vi "CleanReplyPi.vi"(10 "text read":string, 11 "Console in":string) -> (3 "String out":string)   [LabVIEW 2019]
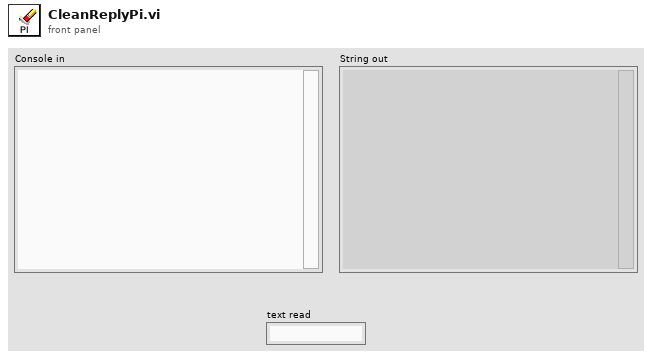
[diagram p1: front panel]
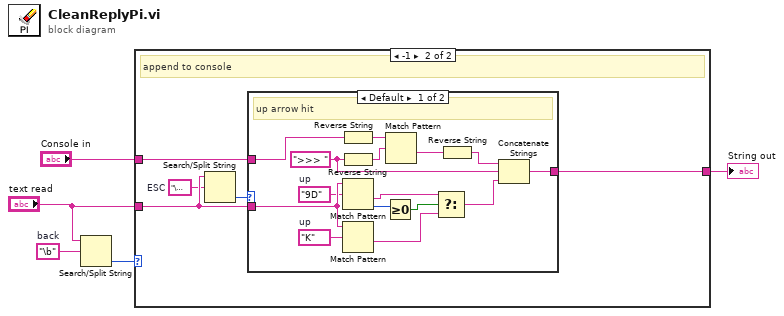
[diagram p0: block diagram]
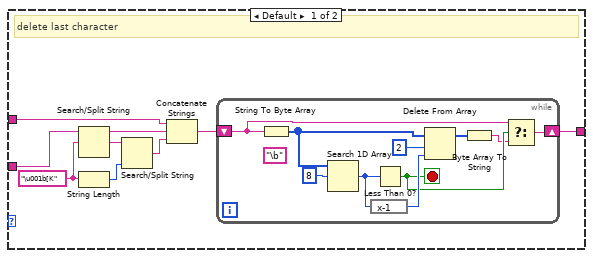
[diagram p2: hidden frame]
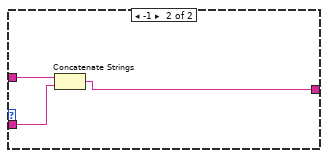
[diagram p3: hidden frame]
diagram:
  w2 = "\b"  # back
  n1 = Search/Split String(string="text read", search string/char (-)=w2) -> (offset of match=w5:i32)  [unwired: 1 in, 2 out]
  n2 = case shown="-1" w5 {
    tunnel: "text read" -> [w12 w27]
    tunnel: "Console in" -> [w14 w29]
    tunnel: [w13 w28] -> w1
    frame Default {
      w9 = "\u001b[K"
      # "delete last character"
      n3 = Search/Split String(string=w12, search string/char (-)=w9) -> (substring before match=w6:string, match + rest of string=w8:string)  [unwired: 1 in, 1 out]
      n4 = String Length(string=w9) -> (length=w10:i32)
      n5 = Search/Split String(string=w8, offset (0)=w10) -> (match + rest of string=w11:string)  [unwired: 1 in, 2 out]
      n6 = Concatenate Strings(w14, w6, w11) -> (w7:string)
      n7 = while {
        shift-right: [w15] -> w13
        shift-left: w7 -> [w17]
        stop <- w18 stop-if-true
        (unwired) "\b"
        n8 = String To Byte Array(string=w17) -> (unsigned byte array=w23:u8[])
        n9 = Search 1D Array(1D array=w23, element=u8 8) -> (index of element=w19:i32)  [unwired: 1 in]
        n10 = expression code="x-1"(w19) -> (w21:i32)
        n11 = Less Than 0?(x=w19) -> (x < 0?=w18:bool)
        n12 = Delete From Array(array=w23, length=2, index=w21) -> (array with subset deleted=w20:u8[])  [unwired: 1 out]
        n13 = Byte Array To String(unsigned byte array=w20) -> (string=w16:string)
        n14 = Select(t=w17, s=w18, f=w16) -> (s? t:f=w15:string)
      }
    }
    frame -1 {
      w25 = "\u001b"  # ESC
      # "append to console"
      n15 = Search/Split String(string=w27, search string/char (-)=w25) -> (offset of match=w26:i32)  [unwired: 1 in, 2 out]
      n16 = case shown="Default" w26 {
        tunnel: w29 -> [w44 w47]
        tunnel: [w43 w46] -> w28
        tunnel: w27 -> [w42 w45]
        frame Default {
          w36 = "K"  # up
          w35 = "9D"  # up
          w30 = ">>> "
          # "up arrow hit"
          n17 = Reverse String(1:w44) -> (0:w32:string)
          n18 = Reverse String(1:w30) -> (0:w34:string)
          n19 = Match Pattern(string=w42, regular expression=w35) -> (after substring=w39:string, offset past match=w37:i32)  [unwired: 1 in, 2 out]
          n20 = Match Pattern(string=w42, regular expression=w36) -> (after substring=w40:string)  [unwired: 1 in, 3 out]
          n21 = Greater Or Equal To 0?(x=w37) -> (x >= 0?=w38:bool)
          n22 = Match Pattern(string=w32, regular expression=w34) -> (after substring=w33:string)  [unwired: 1 in, 3 out]
          n23 = Select(t=w39, s=w38, f=w40) -> (s? t:f=w41:string)
          n24 = Reverse String(1:w33) -> (0:w31:string)
          n25 = Concatenate Strings(w31, w30, w41) -> (w43:string)
        }
        frame -1 {
          n26 = Concatenate Strings(w47, w45) -> (w46:string)
        }
      }
    }
  }
  "String out" <- w1
